vi "Error_2layerOutX_1layerOutX_FPGA.vi"(1 "Array_target_ox":fxp<+/-,32,8>[](array[numeric])=[0.0, 0.0, 0.0, 0.0, 0.0, 0.0, 0.0, 0.0], 2 "Array_Out_ox":fxp<+/-,32,8>[](array[numeric])=[0.0, 0.0, 0.0, 0.0, 0.0, 0.0, 0.0, 0.0], 3 "Array_2layer_Weights_at_Index_hx":fxp<+/-,32,8>[](array[numeric])=[0.0, 0.0, 0.0, 0.0, 0.0, 0.0, 0.0, 0.0]) -> (0 "Err_outX":fxp<+/-,32,8>)   [LabVIEW 2016]
uses:
  <vilib>/rvi/Emulation/niFpgaGetClockAttributes.vi
  <vilib>/rvi/Emulation/niFpgaSctlEmulationGetInTimedLoop.vi
  <vilib>/rvi/Emulation/niFpgaEmulationReportErrorSimple.vi
  <vilib>/rvi/Emulation/niFpgaCriticalErrorInLSC.vi
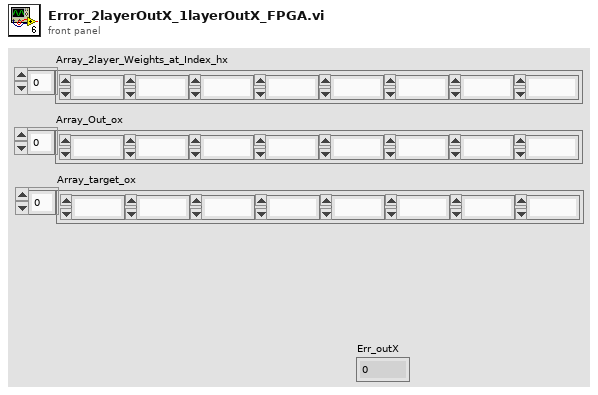
[diagram p1: front panel]
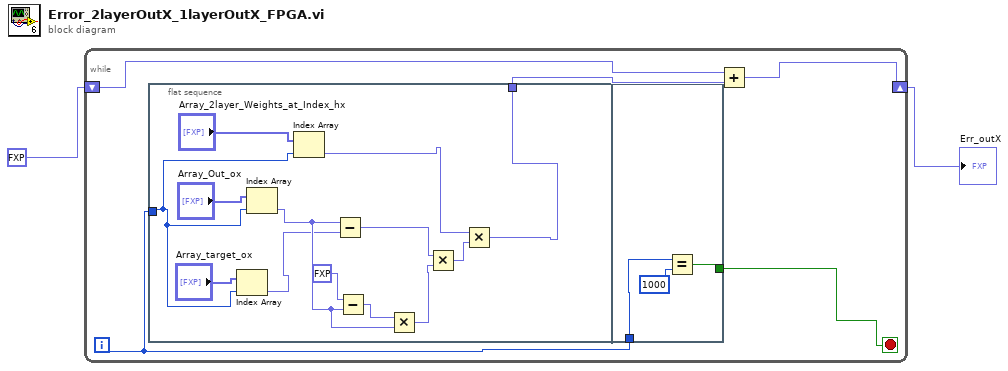
[diagram p0: block diagram]
diagram:
  n1 = while {
    shift-right: [w5] -> w1
    shift-left: fxp<+/-,32,8> 0.0 -> [w6]
    i -> [w4]
    stop <- w3 stop-if-true
    n2 = flat-sequence {
      tunnel: [w13] -> w7
      tunnel: w4 -> [w9]
      tunnel: w4 -> [w22]
      tunnel: [w21] -> w3
      frame #0 {
        n3 = Index Array(array="Array_target_ox", index=w9) -> (element=w8:fxp<+/-,32,8>)
        n4 = Index Array(array="Array_Out_ox", index=w9) -> (element=w11:fxp<+/-,32,8>)
        n5 = Index Array(array="Array_2layer_Weights_at_Index_hx", index=w9) -> (element=w14:fxp<+/-,32,8>)
        n6 = Subtract(x=w11, y=w8) -> (x-y=w18:fxp<+/-,33,9>)
        n7 = Subtract(x=fxp<+,32,8> 1.0, y=w11) -> (x-y=w19:fxp<+/-,34,10>)
        n8 = Multiply(x=w19, y=w11) -> (x*y=w17:fxp<+/-,32,8>)
        n9 = Multiply(x=w18, y=w17) -> (x*y=w16:fxp<+/-,64,16>)
        n10 = Multiply(x=w14, y=w16) -> (x*y=w13:fxp<+/-,32,8>)
      }
      frame #1 {
        n11 = Equal?(x=w22, y=1000) -> (x = y?=w21:bool)
      }
    }
    n12 = Add(x=w6, y=w7) -> (x+y=w5:fxp<+/-,32,8>)
  }
  "Err_outX" <- w1
